vi "Set Protection Configuration.vi"(8 "error in":errorcluster, 10 "Selected Channels":T1 {"Input Channels"."Node Ref" format="%.0x"}, 11 "Parent Ref":T3=18446744073709551615 format="%.0x") -> (0 "error out":errorcluster, 3 "Parent Ref Out":T3=18446744073709551615 format="%.0x")   [LabVIEW 2015, in "Protection and Rolling Counter Addon System Explorer.lvlib"]
uses:
  Protection and Rolling Counter Addon System Explorer.lvlib
  <vilib>/NI Veristand/Custom Device API/Custom Device Item Ref.ctl
  Types/Protection Signal Settings.ctl
  Types/Protection Signal Linked Channels.ctl
  Shared/Types/Protection Type.ctl
  <vilib>/NI Veristand/Custom Device API/Set Item Property (Dependent Node Pointer).vi
  Shared/SubVIs/GUID Lookup.vi
  <vilib>/NI Veristand/Custom Device API/Set Item Property (String Array).vi
  <vilib>/NI Veristand/Custom Device API/Set Item Property (U32).vi
  <vilib>/NI Veristand/Custom Device API/Custom Device API.lvlib
  Shared/Protection and Rolling Counter Addon Shared.lvlib
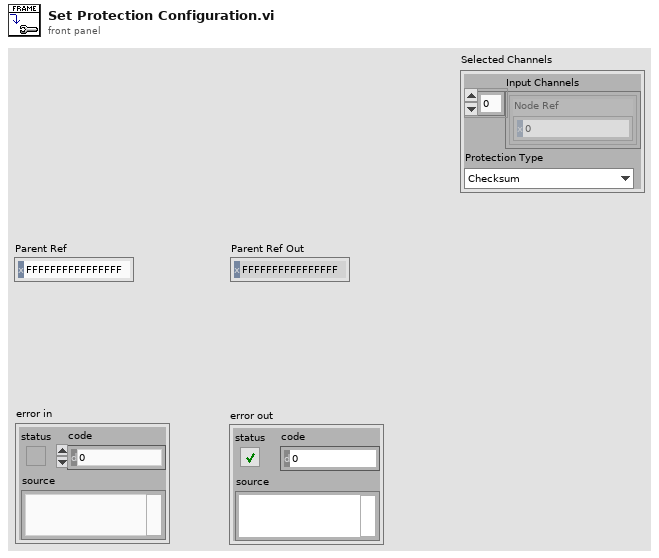
[diagram p1: front panel]
types:
  T1 = typedef "Protection and Rolling Counter Addon System Explorer.lvlib/Protection Signal Settings.ctl" = cluster{"Input Channels":T2[], "Protection Type":T4}
  T2 = typedef "Protection and Rolling Counter Addon System Explorer.lvlib/Protection Signal Linked Channels.ctl" = cluster{"Node Ref":T3}
  T3 = typedef "Custom Device API.lvlib/Custom Device Item Ref.ctl" = u64
  T4 = typedef "Protection and Rolling Counter Addon Shared.lvlib/Protection Type.ctl" = enum16{"Checksum", "CRC", "None (Counter Only)"}
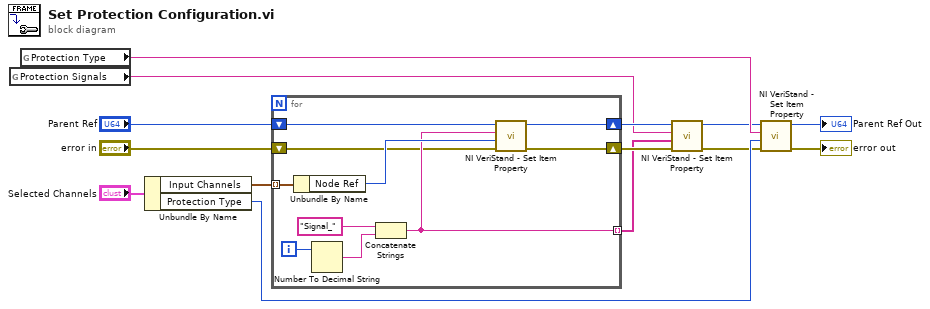
[diagram p0: block diagram]
diagram:
  n1 = global read "GUID Lookup.vi" "Protection Signals"() -> (w7:string)
  n2 = global read "GUID Lookup.vi" "Protection Type"() -> (w6:string)
  n3 = Unbundle By Name("Selected Channels") -> ("Input Channels"=w11:T2[], "Protection Type"=w3:T4)
  n4 = for {
    tunnel: w11 -> [w21] mode=indexing
    tunnel: [w19] -> w8 mode=indexing
    shift-right: [w17] -> w10
    shift-left: "error in" -> [w18]
    shift-right: [w15] -> w9
    shift-left: "Parent Ref" -> [w16]
    i -> [w23]
    n5 = Unbundle By Name(w21) -> ("Node Ref"=w20:T3)
    n6 = Number To Decimal String(number=w23) -> (decimal integer string=w22:string)  [unwired: 1 in]
    n7 = Concatenate Strings("Signal_" ("string"), w22) -> (w19:string)
    n8 = call-poly <vilib>:"NI VeriStand - Set Item Property.vi"("error in (no error)"=w18, "Dependent Node Ref"=w20, "Property Name"=w19, "Item Ref in"=w16) -> ("error out"=w17:errorcluster, "Item Ref out"=w15:T3)  [unwired: 5 in, 1 out]
  }
  n9 = call-poly <vilib>:"NI VeriStand - Set Item Property.vi"("error in (no error)"=w10, "Value"=w8, "Property Name"=w7, "Item Ref in"=w9) -> ("error out"=w1:errorcluster, "Item Ref out"=w4:T3)  [unwired: 5 in, 1 out]
  n10 = call-poly <vilib>:"NI VeriStand - Set Item Property.vi"("error in (no error)"=w1, "Value"=w3, "Property Name"=w6, "Item Ref in"=w4) -> ("error out"=→"error out":errorcluster, "Item Ref out"=→"Parent Ref Out":T3)  [unwired: 5 in, 1 out]
